vi "Wait For Acquisition Time Out.vi"(11 "iTimeOutMs":i32) -> (3 "function return":u32)   [LabVIEW 2018, in "AndorSDK.lvlib"]
doc: "EXPNETTYPE unsigned int WINAPI WaitForAcquisitionTimeOut(int iTimeOutMs);"
uses:
  AndorSDK.lvlib
  ATMCD32D.dll
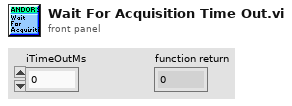
[diagram p1: front panel]
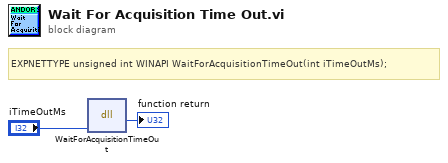
[diagram p0: block diagram]
diagram:
  # "EXPNETTYPE unsigned int WINAPI WaitForAcquisitionTimeOut(int iTimeOutMs);"
  n1 = dll-call lib="PTH2babs E\nPersönliches02 - Arbeit03-HiwijobsLabviewCodelibANDOR\tAndor SDK\nATMCD32D.*" fn="WaitForAcquisitionTimeOut"("iTimeOutMs"="iTimeOutMs") -> (→"function return":u32)  [unwired: 4 in, 2 out]
